vi "Modell.vi"(8 "Winkel_t0":dbl, 9 "Winkelg._t0":dbl, 10 "output (Eingang)":dbl, 11 "Position_t0":dbl) -> (0 "Winkelgesch":dbl, 1 "Winkel":dbl, 2 "Geschwindigkeit":dbl, 3 "Position":dbl)   [LabVIEW 2014]
uses:
  <vilib>/Simulation/Implementation/Shared/SIMSCR Execution Mode.ctl
  <vilib>/Simulation/Scripting/Companion Diagram/SimConfigNode/SimParams.ctl
  <vilib>/Simulation/Scripting/Companion Diagram/SimConfigNode/_simSolvers.ctl
  <vilib>/Simulation/Param Hierarchy/Typedefs/SIMPH Param Control Actions.ctl
  <vilib>/Simulation/Implementation/Shared/SIM limit type.ctl
  <vilib>/Simulation/Implementation/Shared/NILVSim_ParamChanged.vi
  <vilib>/Simulation/Implementation/Shared/NILVSIM_BeginStep.vi
  <vilib>/Simulation/ContinuousLinear/Implementation/NILVSim Integrator new.llb/SIM Integrator distributor (scalar).vi
  <vilib>/Simulation/ContinuousLinear/Implementation/NILVSim Integrator new.llb/SIM Integrator collector (scalar).vi
  <vilib>/Simulation/Implementation/Shared/NILVSim_Manager.vi
  <vilib>/Utility/error.llb/Clear Errors.vi
  <vilib>/Simulation/Implementation/Shared/NILVSim_FinalizeModel.vi
  <vilib>/Simulation/Implementation/Shared/SIM Unbundle Sim Info.vi
  <vilib>/Simulation/Implementation/Shared/SIMSH Read Queue.vi
  <vilib>/Simulation/Implementation/Shared/NILVSim_Initialize.vi
  <vilib>/Simulation/Utility/Implementation/NILVSim Get Time and IsAcceptedStep.vi
  <vilib>/Simulation/Implementation/Shared/NILVSim_GetModelError.vi
  <vilib>/Simulation/Implementation/Shared/SIM SimErrorHandler.vi
  <vilib>/Simulation/Implementation/Shared/SIM Bundle Sim Info.vi
  <vilib>/Simulation/Scripting/Companion Diagram/SimConfigNode/SimDog.xnode
  <vilib>/Simulation/ContinuousLinear/Implementation/NILVSim Integrator new.llb/SIM Integrator (scalar).vi
  <vilib>/Simulation/Implementation/XNodeFramework/SimXNode/SimX.xnode
  <vilib>/Simulation/Implementation/Shared/NI_SIM_Implementation.lvlib
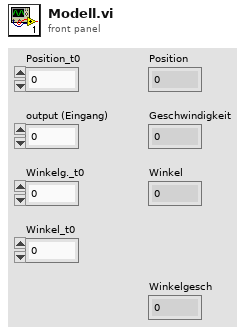
[diagram p1: front panel]
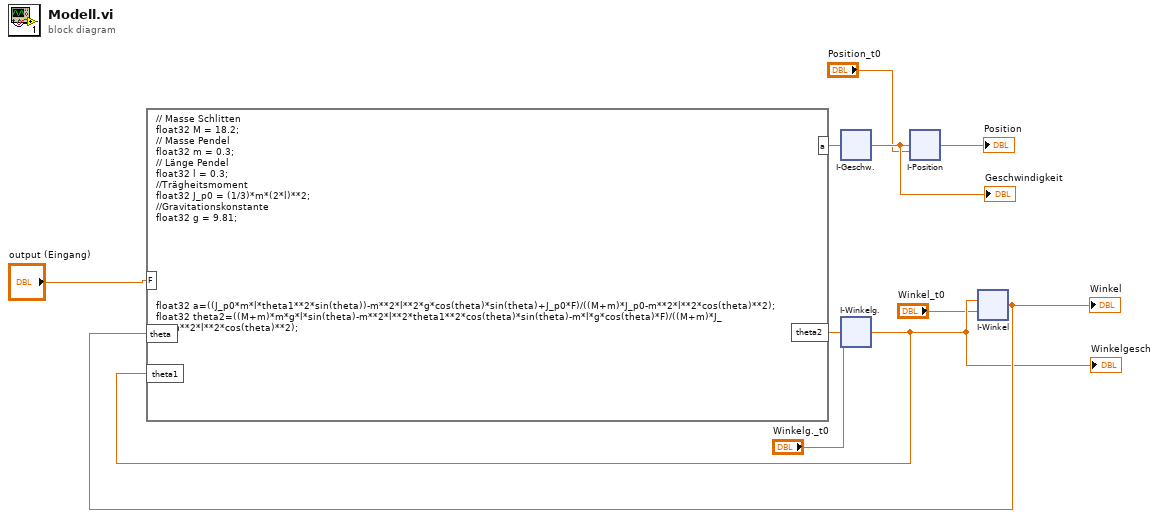
[diagram p0: block diagram]
diagram:
  n1 = formula code="// Masse Schlitten\nfloat32 M = 18.2;\n// Masse Pendel\nfloat32 m = 0.3;\n// Länge Pendel\nfloat32 l = 0.3;\n//Trägheitsmoment\nfloat32 J_p0 = (1/3)*m*(2*l)**2;\n//Gravitationskonstante\nfloat32 g = 9.81;\n\n\n\n\n\n\n\nfloat32 a=((J_p0*m*l*theta1**2*sin(theta))-m**2*l**2*g*cos(theta)*sin(theta)+J_p0*F)/((M+m)*J_p0-m**2*l**2*cos(theta)**2);\nfloat32 theta2=((M+m)*m*g*l*sin(theta)-m**2*l**2*theta1**2*cos(theta)*sin(theta)-m*l*g*cos(theta)*F)/((M+m)*J_p0-m**2*l**2*cos(theta)**2);" ("Formelknoten")("theta"=w7, "theta1"=w6, "F"="output (Eingang)") -> ("a"=w4:sgl, "theta2"=w3:sgl)
  n2 = xnode "I-Geschw."("input"=w4) -> ("output"=w8:dbl)  [unwired: 9 in, 2 out]
  "Geschwindigkeit" <- w8
  n3 = xnode "I-Winkelg."("input"=w3, "initial condition"="Winkelg._t0") -> ("output"=w6:dbl)  [unwired: 8 in, 2 out]
  "Winkelgesch" <- w6
  n4 = xnode "I-Position"("input"=w8, "initial condition"="Position_t0") -> ("output"=→"Position":dbl)  [unwired: 8 in, 2 out]
  n5 = xnode "I-Winkel"("input"=w6, "initial condition"="Winkel_t0") -> ("output"=w7:dbl)  [unwired: 8 in, 2 out]
  "Winkel" <- w7
